vi "HDF5_append-dataset-Test8vi.vi"() -> ()   [LabVIEW 2018]
uses:
  <vilib>/addons/h5labview2/file/H5F.lvlib
  <vilib>/addons/h5labview2/file/H5Fmode.ctl
  <vilib>/addons/h5labview2/dataset/H5D.lvlib
  HDF5/HDF5_ToneInfoClust.ctl
  <vilib>/addons/h5labview2/dataset/H5Dwrite.llb/H5Dwrite.xnode
  <vilib>/addons/h5labview2/space/H5S.lvlib
  <vilib>/addons/h5labview2/base/H5Equery.vi
  HDF5/lib_path_mod_20200519.vi
  <vilib>/addons/h5labview2/dataset/H5Dread.llb/H5Dread.xnode
  <vilib>/addons/h5labview2/group/H5G.lvlib
  <vilib>/addons/h5labview2/base/hid_t_renamed.ctl
  <vilib>/addons/h5labview2/base/h5o_type.ctl
panel:
  out "names 2":string[](array[string])
  out "types 2":T1[](array[typedef])
  out "types":T1[](array[typedef])
  out "names":string[](array[string])
  in  "Zoom":dbl[](array[numeric])
  out "Tone2":T2[](array[typedef])
  out "Tone1":T2[](array[typedef])
  out "ms/append":dbl
  out "timer (ms)":u32
  out "progress":i32(slide)=9999 scale=0.0..10.0
  in  "repetitions":i32=10
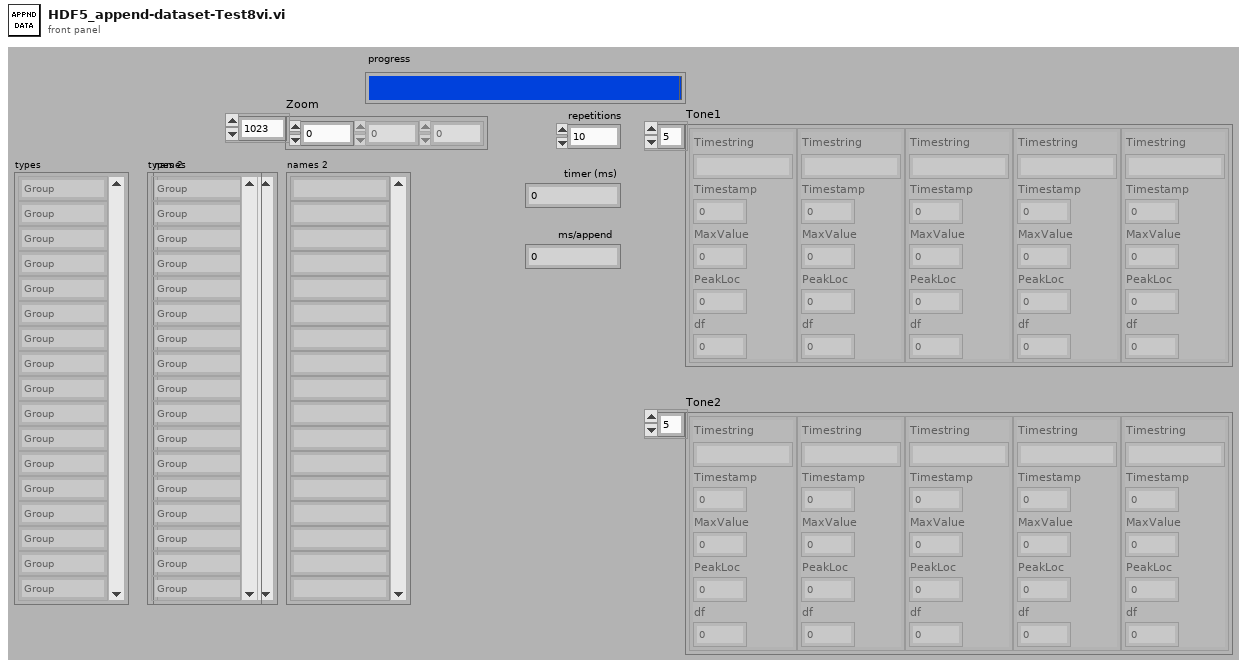
[diagram p1: front panel]
types:
  T1 = typedef "h5o_type.ctl" = enum8{"Group", "Dataset", "Named type"}
  T2 = typedef "HDF5_ToneInfoClust.ctl" = cluster{"Timestring":string, "Timestamp":dbl, "MaxValue":dbl, "PeakLoc":dbl, "df":dbl}
  T3 = typedef "H5F.lvlib/H5Fmode.ctl" = enum16{"read-only", "read-write", "overwrite", "create new", "open or create"}
  T4 = typedef "hid_t.ctl" = i32
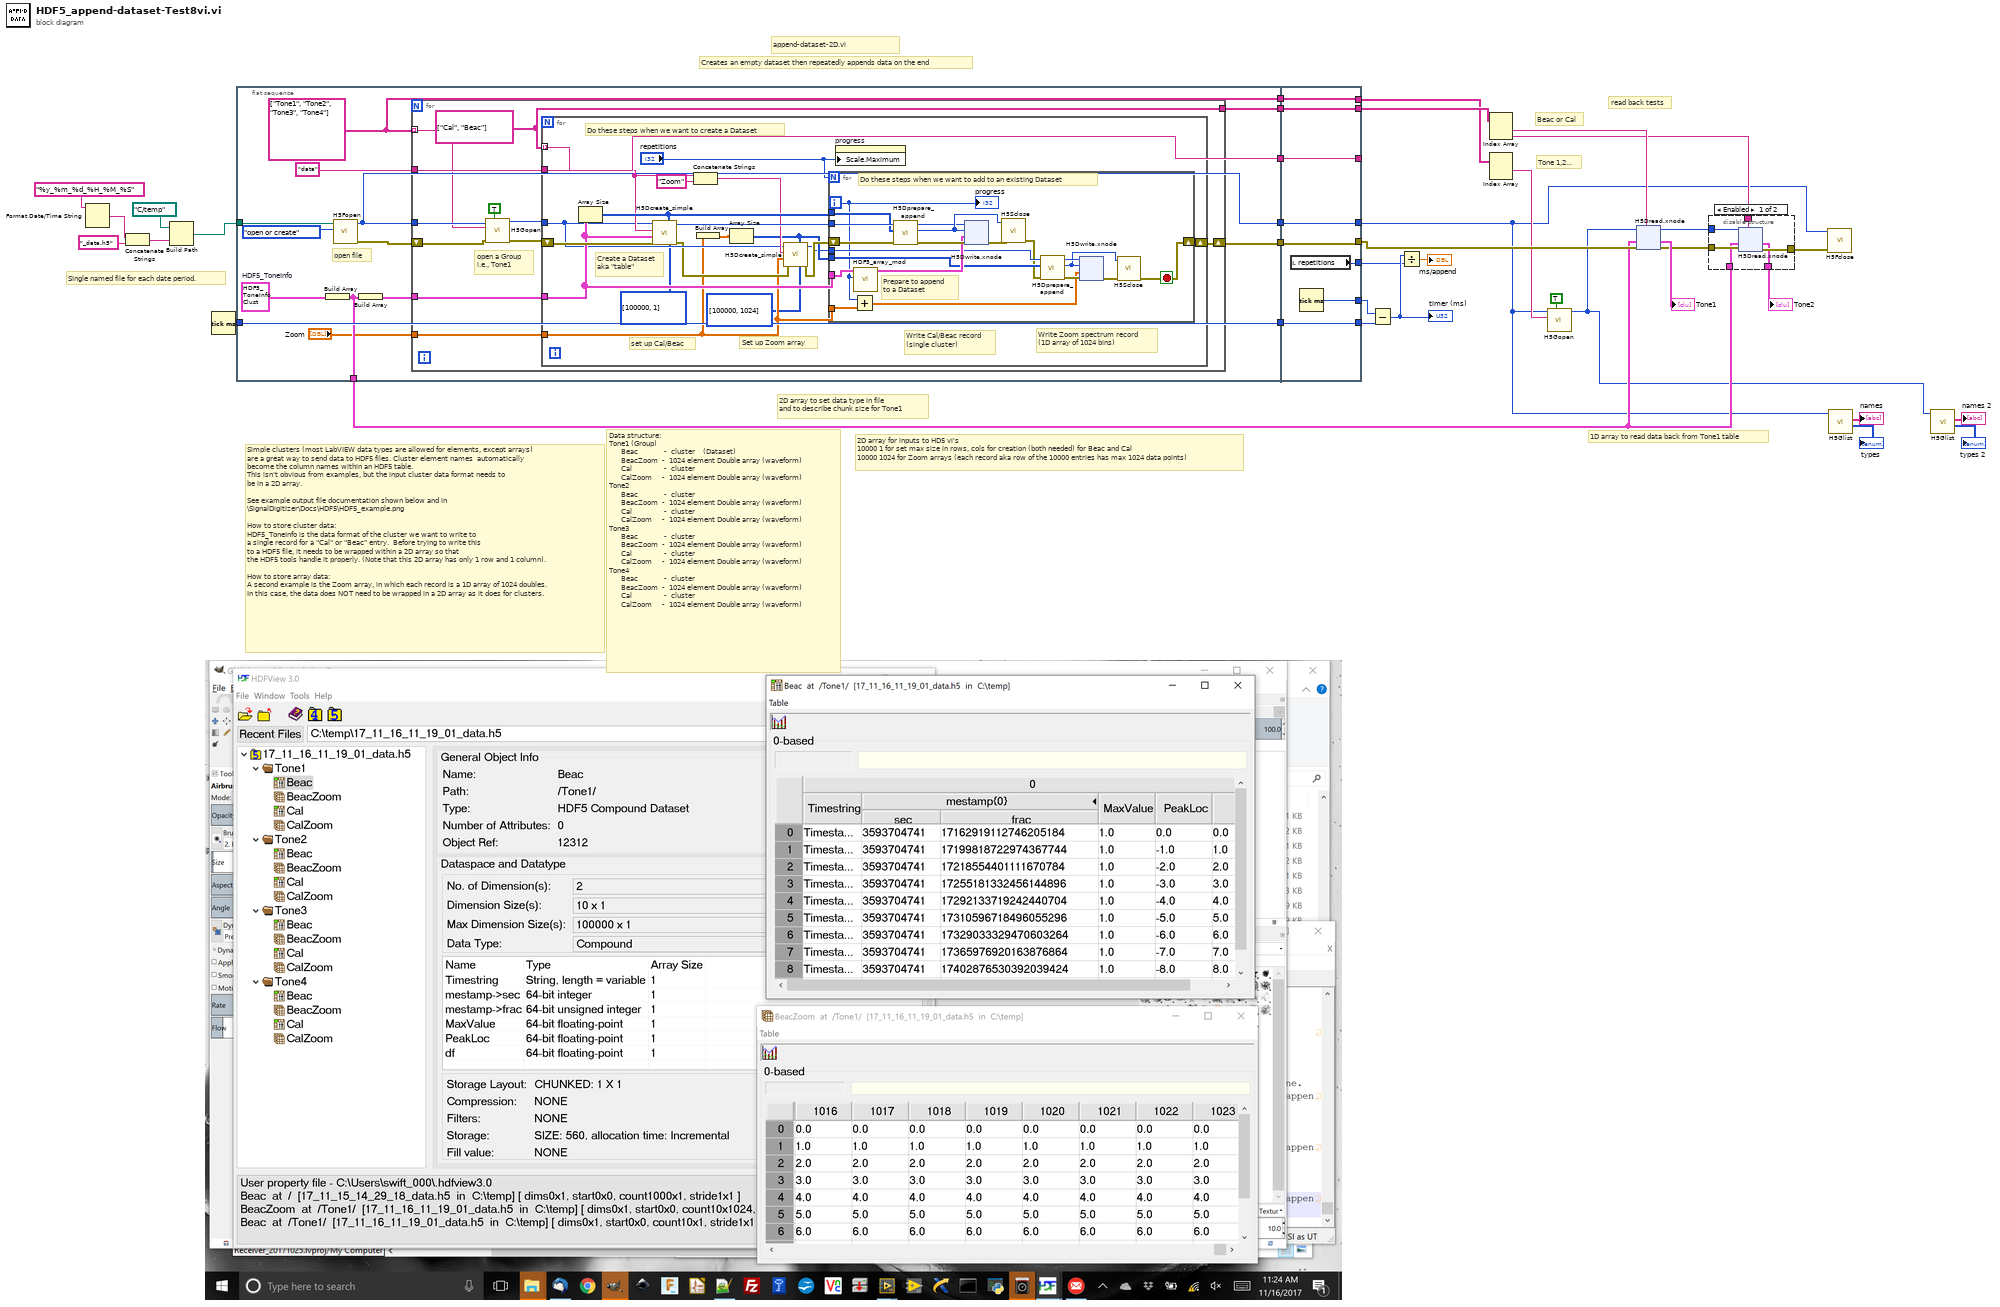
[diagram p0: block diagram]
diagram:
  # "Data structure:\nTone1 (Group)                                       \n      Beac             -  cluster    (Dataset)\n      BeacZoom  -  1024 element Double array (waveform) \n      Cal                -  cluster\n      CalZoom     -  1024 element Double array (waveform) \nTone2\n      Beac             -  cluster\n      BeacZoom  -  1024 element Double array (waveform) \n      Cal                -  cluster\n      CalZoom     -  1024 element Double array (waveform) \nTone3\n      Beac             -  cluster\n      BeacZoom  -  1024 element Double array (waveform) \n      Cal                -  cluster\n      CalZoom     -  1024 element Double array (waveform) \nTone4\n      Beac             -  cluster\n      BeacZoom  -  1024 element Double array (waveform) \n      Cal                -  cluster\n      CalZoom     -  1024 element Double array (waveform)"
  # "Simple clusters (most LabVIEW data types are allowed for elements, except arrays) \nare a great way to send data to HDF5 files. Cluster element names  automatically\nbecome the column names within an HDF5 table.\nThis isn't obvious from examples, but the input cluster data format needs to \nbe in a 2D array.\n\nSee example output file documentation shown below and in\n\\SignalDigitizer\\Docs\\HDF5\\HDF5_example.png\n\nHow to store cluster data:\nHDF5_ToneInfo is the data format of the cluster we want to write to \na single record for a \"Cal\" or \"Beac\" entry.  Before trying to write this \nto a HDF5 file, it needs to be wrapped within a 2D array so that \nthe HDF5 tools handle it properly. (Note that this 2D array has only 1 row and 1 column).\n\nHow to store array data:\nA second example is the Zoom array, in which each record is a 1D array of 1024 doubles.\nIn this case, the data does NOT need to be wrapped in a 2D array as it does for clusters."
  # "Tone 1,2..."
  # "Beac or Cal"
  # "read back tests"
  # "2D array to set data type in file\nand to describe chunk size for Tone1"
  # "1D array to read data back from Tone1 table"
  # "2D array for inputs to HD5 vi's\n10000 1 for set max size in rows, cols for creation (both needed) for Beac and Cal\n10000 1024 for Zoom arrays (each record aka row of the 10000 entries has max 1024 data points)"
  # "Single named file for each date period."
  # "Creates an empty dataset then repeatedly appends data on the end"
  # "append-dataset-2D.vi"
  n1 = Format Date/Time String(time format string (%c)="%y_%m_%d_%H_%M_%S") -> (date/time string=w27:string)  [unwired: 2 in]
  n2 = Concatenate Strings(w27, "_data.h5" ("string")) -> (w29:string)
  n3 = Build Path(base path=path "C:/temp", name or relative path=w29) -> (appended path=w25:path)
  n4 = Tick Count (ms)() -> (millisecond timer value=w37:u32)
  n5 = flat-sequence {
    tunnel: w37 -> [w49]
    tunnel: [w49] -> w36
    tunnel: w25 -> [w48]
    tunnel: [w40] -> w24
    tunnel: [w45] -> w23
    tunnel: [w44] -> w12
    tunnel: [w43] -> w21
    tunnel: [w42] -> w19
    tunnel: [w38] -> w9
    tunnel: w36 -> [w144]
    tunnel: [w145] -> w35
    tunnel: [w144] -> w34
    tunnel: [w143] -> w32
    tunnel: [w142] -> w6
    tunnel: w24 -> [w142]
    tunnel: [w141] -> _
    tunnel: w23 -> [w141]
    tunnel: [w140] -> w20
    tunnel: w21 -> [w140]
    tunnel: w19 -> [w139]
    tunnel: [w139] -> w17
    tunnel: [w138] -> w8
    tunnel: w9 -> [w138]
    frame #0 {
      w38 = string[] ["Tone1", "Tone2", "Tone3", "Tone4"]
      w47 = T2 {"Timestring"="Timestamp string goes here", "Timestamp"=0.0, "MaxValue"=0.0, "PeakLoc"=0.0, "df"=0.0}  # HDF5_ToneInfo
      w45 = "data" ("name")
      # "open file"
      n6 = Build Array(w47) -> (w44:T2[])
      n7 = call <vilib>:"H5Fopen.vi"("mode (read-only)"=H5Fmode."open or create" ("mode"), "path"=w48) -> ("error out"=w39:errorcluster, "ref out"=w40:T4)  [unwired: 8 in]
      n8 = Build Array(w44) -> (w46:T2[][])
      n9 = for {
        tunnel: w46 -> [w61]
        tunnel: w45 -> [w60]
        tunnel: [w58] -> w42
        tunnel: "Zoom" -> [w57]
        tunnel: w40 -> [w56]
        shift-right: [w59] -> w43
        shift-left: w39 -> [w52]
        tunnel: w38 -> [w51] mode=indexing
        w58 = string[] ["Cal", "Beac"]
        # "open a Group\ni.e., Tone1"
        n10 = call <vilib>:"H5Gopen.vi"("create? (F)"=TRUE, "error in (no error)"=w52, "name"=w51, "ref in"=w56) -> ("error out"=w53:errorcluster, "group out"=w54:T4)  [unwired: 6 in]
        n11 = for {
          tunnel: w61 -> [w76]
          tunnel: w54 -> [w70]
          tunnel: w60 -> [_]
          shift-right: [w74] -> w59
          shift-left: w53 -> [w78]
          tunnel: w58 -> [w73] mode=indexing
          tunnel: w57 -> [w63]
          # "Do these steps when we want to create a Dataset"
          # "Create a Dataset\naka \"table\""
          # "Write Zoom spectrum record\n(1D array of 1024 bins)"
          # "Write Cal/Beac record\n(single cluster)"
          # "Set up Zoom array"
          # "set up Cal/Beac"
          n12 = Array Size(array=w76) -> (size(s)=w75:i32[])
          n13 = call <vilib>:"H5Dcreate_simple.vi"("max size"=u64[] [100000, 1], "chunk size"=w75, "error in (no error)"=w78, "type in"=w76, "name"=w73, "ref in"=w70) -> ("error out"=w67:errorcluster, "dset out"=w79:T4)  [unwired: 4 in]
          n14 = Concatenate Strings(w73, "Zoom" ("string")) -> (w71:string)
          n15 = Build Array(w63) -> (w69:dbl[][])
          n16 = Array Size(array=w69) -> (size(s)=w65:i32[])
          n17 = call <vilib>:"H5Dcreate_simple.vi"("max size"=u64[] [100000, 1024], "chunk size"=w65, "error in (no error)"=w67, "type in"=w63, "name"=w71, "ref in"=w70) -> ("error out"=w66:errorcluster, "dset out"=w64:T4)  [unwired: 4 in]
          n18 = for {
            N: "repetitions" -> [_]
            shift-right: [w83] -> w74
            shift-left: w66 -> [w96]
            tunnel: w75 -> [w97]
            tunnel: w79 -> [w98]
            tunnel: w76 -> [w92]
            tunnel: w65 -> [w90]
            tunnel: w64 -> [w89]
            tunnel: w63 -> [w81]
            i -> [w82]
            stop <- w83 stop-if-true
            # "Do these steps when we want to add to an existing Dataset"
            # "Prepare to append\nto a Dataset"
            n19 = Add(x=w82, y=w81) -> (x+y=w80:dbl[])
            n20 = call "HDF5_array_mod.vi"("delta"=w82, "Array in"=w92) -> ("Array out"=w91:T2[][])  [unwired: 9 in]
            n21 = call <vilib>:"H5Dprepare_append.vi"("error in (no error)"=w96, "append dims"=w97, "dset in"=w98) -> ("error out"=w99:errorcluster, "space out"=w94:T4, "dset out"=w93:T4)  [unwired: 5 in, 1 out]
            n22 = xnode "H5Dwrite.xnode"("error in (no error)"=w99, "data"=w91, "file space"=w94, "ref in"=w93) -> ("error out"=w95:errorcluster)  [unwired: 3 in, 2 out]
            n23 = call <vilib>:"H5Sclose.vi"("error in (no error)"=w95, "space in"=w94) -> ("error out"=w88:errorcluster)  [unwired: 9 in]
            n24 = call <vilib>:"H5Dprepare_append.vi"("error in (no error)"=w88, "append dims"=w90, "dset in"=w89) -> ("error out"=w85:errorcluster, "space out"=w86:T4, "dset out"=w87:T4)  [unwired: 5 in, 1 out]
            n25 = xnode "H5Dwrite.xnode"("error in (no error)"=w85, "data"=w80, "file space"=w86, "ref in"=w87) -> ("error out"=w84:errorcluster)  [unwired: 3 in, 2 out]
            n26 = call <vilib>:"H5Sclose.vi"("error in (no error)"=w84, "space in"=w86) -> ("error out"=w83:errorcluster)  [unwired: 9 in]
            "progress" <- w82
          }
          n27 = property on="progress" class="Slide (strict)"("Scale.Maximum"="repetitions") -> ()  [unwired: 2 in, 2 out]
        }
      }
    }
    frame #1 {
      n28 = local read "repetitions"() -> (w143:i32)
      n29 = Tick Count (ms)() -> (millisecond timer value=w145:u32)
    }
  }
  n30 = Subtract(x=w35, y=w34) -> (x-y=w33:u32)
  "timer (ms)" <- w33
  n31 = Divide(x=w33, y=w32) -> (x/y=→"ms/append":dbl)
  n32 = Index Array(array=w17) -> (element #1=w16:string, element #2=w15:string)  [unwired: 2 in]
  n33 = Index Array(array=w8) -> (element #1=w7:string)  [unwired: 2 in, 1 out]
  n34 = call <vilib>:"H5Gopen.vi"("create? (F)"=TRUE, "name"=w7, "ref in"=w6) -> ("group out"=w1:T4)  [unwired: 7 in, 1 out]
  n35 = xnode "H5Dread.xnode"("dataset name (this)"=w16, "error in (no error)"=w20, "default"=w12, "ref in"=w1) -> ("error out"=w14:errorcluster, "data"=→"Tone1":T2[], "ref out"=w18:i32)  [unwired: 2 in, 1 out]
  n36 = disable-structure shown="Enabled" {
    disable-tunnel: w18 -> [w151 _]
    disable-tunnel: w15 -> [w150 _]
    disable-tunnel: w14 -> [w149 w167]
    disable-tunnel: [w148 w167] -> w13
    disable-tunnel: w12 -> [w147 _]
    disable-tunnel: [w146 _] -> w11
    frame Enabled {
      n37 = xnode "H5Dread.xnode"("dataset name (this)"=w150, "error in (no error)"=w149, "default"=w147, "ref in"=w151) -> ("error out"=w148:errorcluster, "data"=w146:T2[])  [unwired: 2 in, 2 out]
    }
    frame Disabled {
    }
  }
  "Tone2" <- w11
  n38 = call <vilib>:"H5Fclose.vi"("error in (no error)"=w13, "ref"=w6) -> ()  [unwired: 9 in, 1 out]
  n39 = call <vilib>:"H5Glist.vi"("ref in"=w6) -> ("types"=→"types":T1[], "names"=→"names":string[])  [unwired: 7 in, 2 out]
  n40 = call <vilib>:"H5Glist.vi"("ref in"=w1) -> ("types"=→"types 2":T1[], "names"=→"names 2":string[])  [unwired: 7 in, 2 out]
